vi "Detector de umbral.vi"() -> ()   [LabVIEW 2016]
uses:
  <vilib>/Analysis/2dsp.llb/1D Cross Correlation (DBL).vi
  <vilib>/Analysis/NI_AALPro.lvlib
  <vilib>/Analysis/NI_AALBase.lvlib
panel:
  out "y(n)":i16
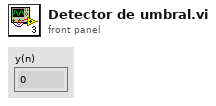
[diagram p1: front panel]
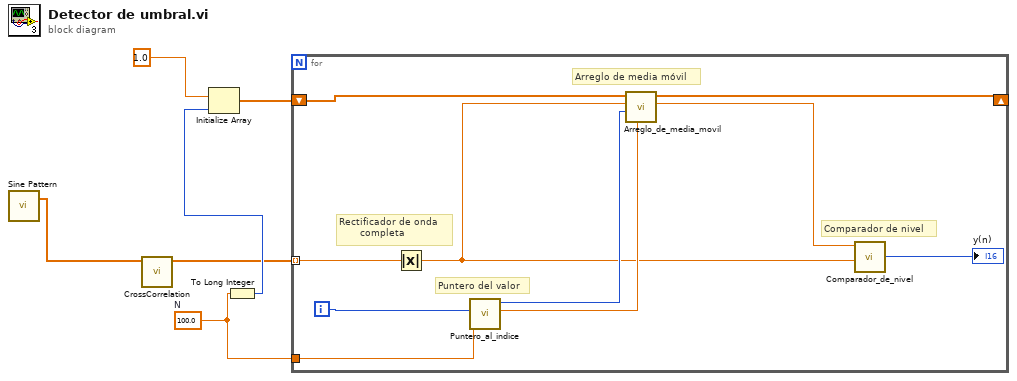
[diagram p0: block diagram]
diagram:
  w4 = 100.0  # N
  n1 = call <vilib>:"Sine Pattern.vi"() -> ("Sinusoidal Pattern"=w1:dbl[])  [unwired: 4 in, 1 out]
  n2 = call-poly <vilib>:"CrossCorrelation.vi"("X"=w1) -> ("Rxy"=w2:dbl[])  [unwired: 9 in, 1 out]
  n3 = To Long Integer(number=w4) -> (32bit integer=w3:i32)
  n4 = Initialize Array(1.0, w3) -> (w5:dbl[])
  n5 = for {
    shift-right: [w12] -> _
    shift-left: w5 -> [w16]
    tunnel: w4 -> [w14]
    tunnel: w2 -> [w7] mode=indexing
    i -> [w15]
    # "Rectificador de onda \n       completa"
    # "Puntero del valor"
    # "Comparador de nivel"
    # "Arreglo de media móvil"
    n6 = Absolute Value(x=w7) -> (abs(x)=w8:dbl)
    n7 = call "Puntero_al_indice.vi"("Numeric in"=w15, "N in"=w14) -> ("N out"=w10:dbl, "Numeric out"=w13:i32)  [unwired: 8 in]
    n8 = call "Arreglo_de_media_movil.vi"("N"=w10, "Numeric 3"=w13, "Numeric in"=w8, "Array in"=w16) -> ("Numeric out"=w11:dbl, "Array out"=w12:dbl[])  [unwired: 6 in]
    n9 = call "Comparador_de_nivel.vi"("Numeric"=w8, "Numeric in"=w11) -> ("Numeric 2"=→"y(n)":i16)  [unwired: 9 in]
  }
